vi "LIMUStatus.vi"(0 "VisaCluster":T1, 11 "error in (no error)":errorcluster) -> (4 "VisaCluster":T1, 6 "Numeric":dbl, 8 "Message Out":string, 15 "error out":errorcluster)   [LabVIEW 2014, in "FH 55.lvlib"]
doc: "Dieses VI gibt den Status der Extremwertausgabe zurück. Die möglichen Ausgaben sind:\n keine Extermwertausgabe \n nur Max-Werte\n Max und Min-Werte\n\nThis VI returns the status of extreme value output. The possible issues are:\n no extreme value output\n only Max values\n Max and Min values"
uses:
  FH 55.lvlib
  TypeDef/VisaCluster.ctl
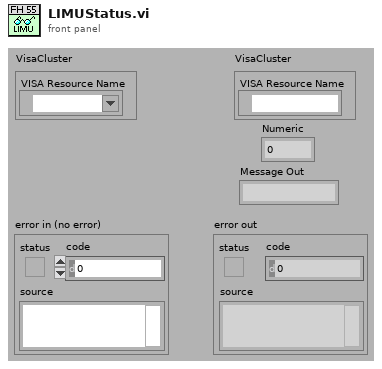
[diagram p1: front panel]
types:
  T1 = typedef "FH 55.lvlib/VisaCluster.ctl" = cluster{"VISA Resource Name":refnum<visa-resource-name>}
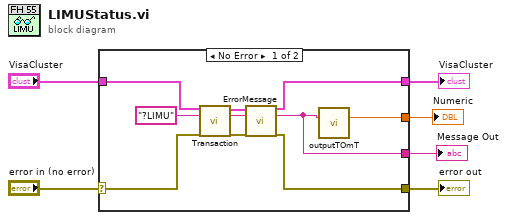
[diagram p0: block diagram]
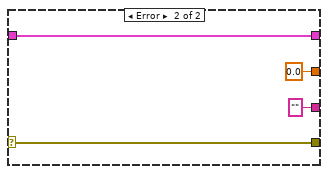
[diagram p2: hidden frame]
diagram:
  n1 = case shown="No Error" "error in (no error)" {
    selector: "error in (no error)" -> [w10 w19]
    tunnel: "VisaCluster" -> [w11 w20]
    tunnel: [w16 w20] -> w3
    tunnel: [w9 w19] -> w4
    tunnel: [w8 0.0 ("Numeric")] -> w2
    tunnel: [w7 "" ("Message Out")] -> w1
    frame No Error {
      n2 = call "Transaction.vi"("VisaCluster"=w11, "Command"="?LIMU", "error in (no error)"=w10) -> ("VisaCluster"=w14:T1, "Answer"=w12:string, "error out"=w15:errorcluster)  [unwired: 9 in, 1 out]
      n3 = call "ErrorMessage.vi"("VisaCluster"=w14, "Message In"=w12, "error in (no error)"=w15) -> ("VisaCluster"=w16:T1, "Message Out"=w7:string, "error out"=w9:errorcluster)  [unwired: 10 in]
      n4 = call "outputTOmT.vi"("Input"=w7) -> ("Numeric"=w8:dbl)  [unwired: 13 in, 1 out]
    }
    frame Error {
    }
  }
  "error out" <- w4
  "VisaCluster" <- w3
  "Numeric" <- w2
  "Message Out" <- w1
